vi "Actor Core.vi"(8 "error in":errorcluster, 11 "Nested in":refnum<class "MicroscopeController.lvclass">) -> (0 "error out":errorcluster, 3 "Actor out":refnum<class "Actor.lvclass">)   [LabVIEW 2020, in "MicroscopeController.lvlib" / "MicroscopeController.lvclass"]
doc: "(<B>Filename</B>: Actor Framework.lvlib:Actor.lvclass:Actor Core.vi)\n\nReceives messages to the actor, reacts to them, and initiates any error handling that may shut the actor down.\n\nDescendant classes may override this VI to append parallel tasks for the actor to complete while it handles messages. Overrides use the Call Parent Method node."
uses:
  MicroscopeController.lvclass
  C:/Program Files/National Instruments/LabVIEW 2020/vi.lib/ActorFramework/Actor/Actor.lvclass
  <vilib>/ActorFramework/Actor/Actor.lvclass
  MicroscopeController.lvclass/MicroscopeController.ctl
  <vilib>/ActorFramework/Actor/Actor.lvclass/Actor.ctl
  <vilib>/ActorFramework/Message Enqueuer/Message Enqueuer.lvclass/Message Enqueuer.ctl
  <vilib>/ActorFramework/Message Enqueuer/Init from Existing Queue.vi
  <vilib>/ActorFramework/Message Enqueuer/Enqueue.vi
  <vilib>/ActorFramework/Stop Msg/Stop Msg.lvclass
  C:/Program Files/National Instruments/LabVIEW 2020/vi.lib/ActorFramework/Message/Message.lvclass
  <vilib>/ActorFramework/Message Priority Queue/Priority Enqueue.vi
  <vilib>/ActorFramework/Message Enqueuer/Message Enqueuer.lvclass
  E:/Development/DevHardSoftware/MicroscopyFramework/ViewController/Microscope Controller/MicroscopeController.lvclass
  E:/Development/DevHardSoftware/MicroscopyFramework/Interface/DataListener/DataListener.lvclass
  E:/Development/DevHardSoftware/MicroscopyFramework/Interface/ErrorHandler/ErrorHandler.lvclass
panel:
  in  "Tab Control":T1(tab)
  out "SystemStatus":string
  # "https://sites.psu.edu/hancocklab/"
  # "Hancock Lab, The Pennsylvania State University.  email: woh1@psu.edu"
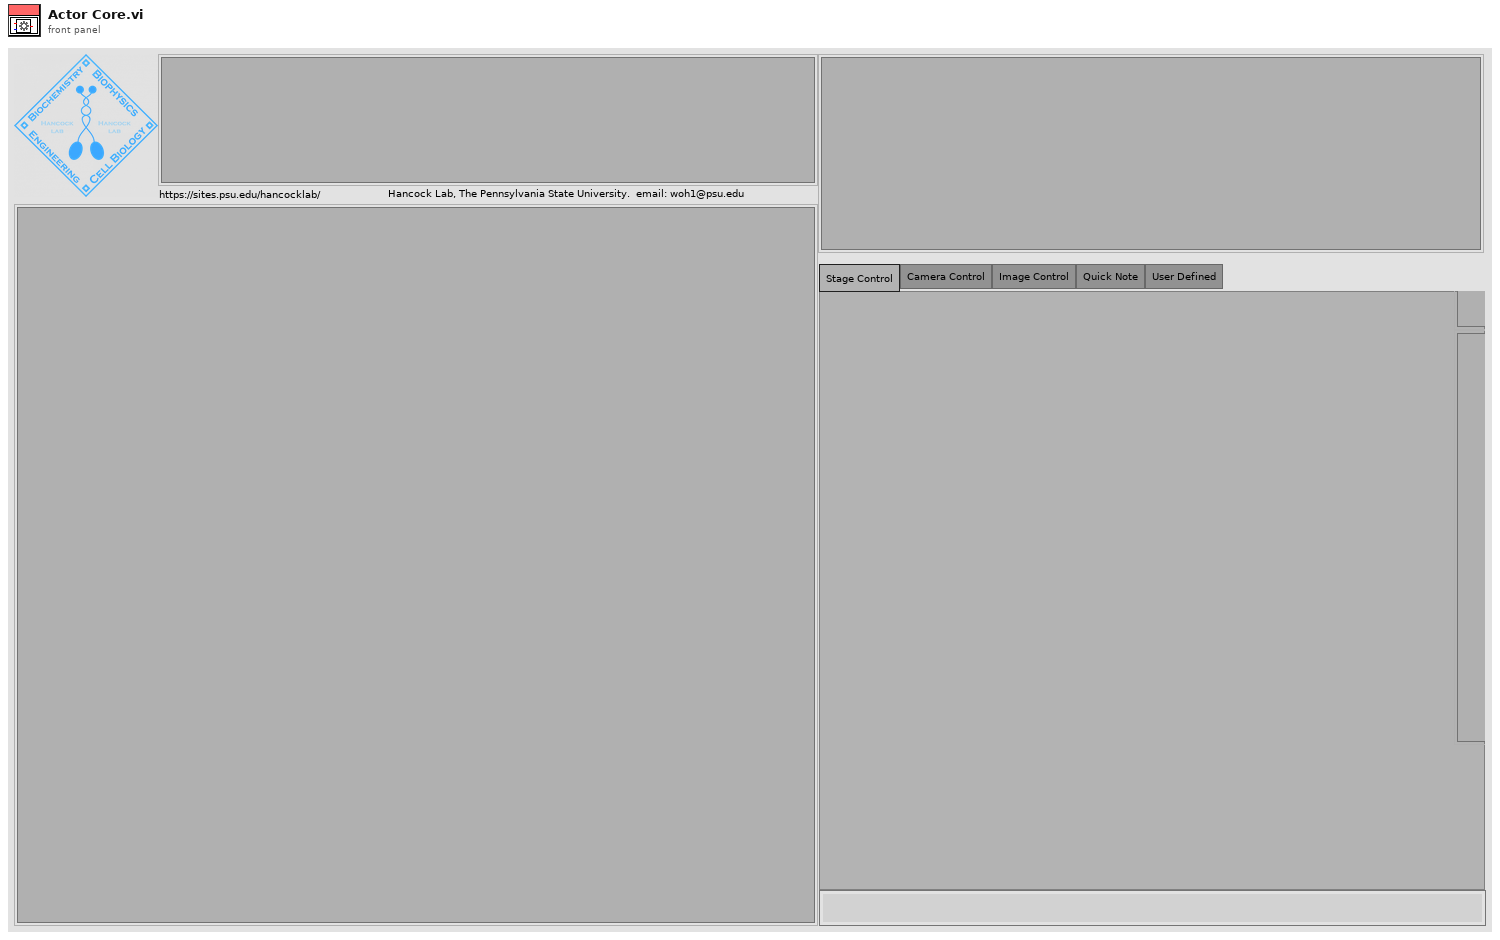
[diagram p1: front panel]
types:
  T1 = enum32{"Stage Control", "Camera Control", "Image Control", "Quick Note", "User Defined"}
  T2 = cluster{"Stop":refnum<user-event>, "SystemStatus":refnum<user-event>}
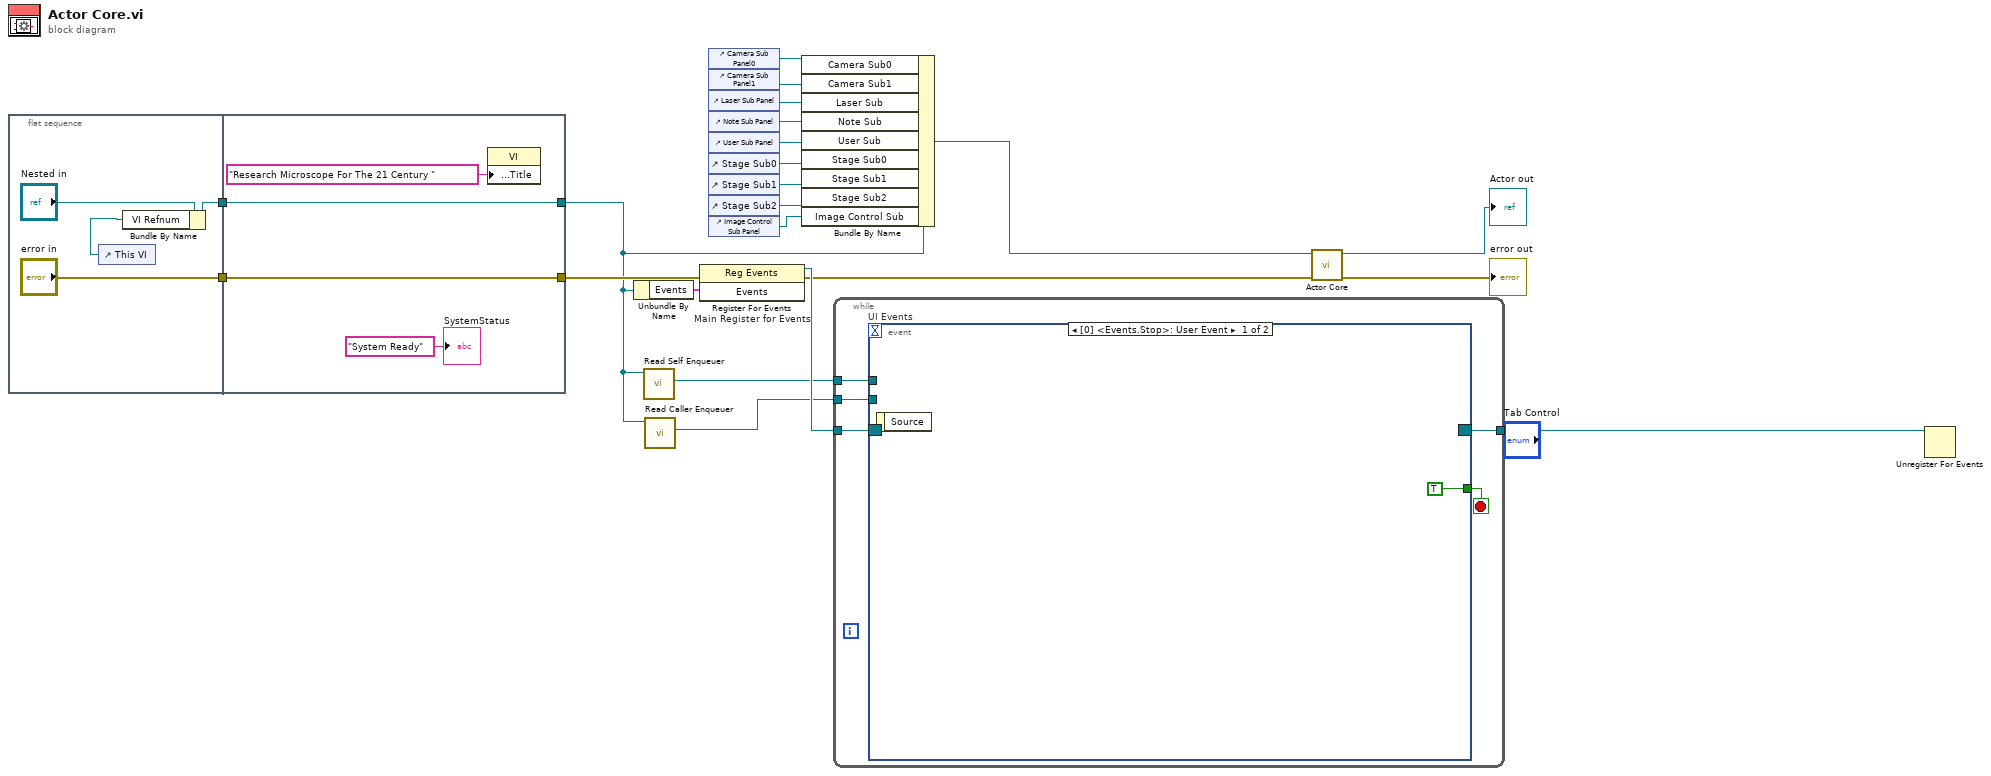
[diagram p0: block diagram]
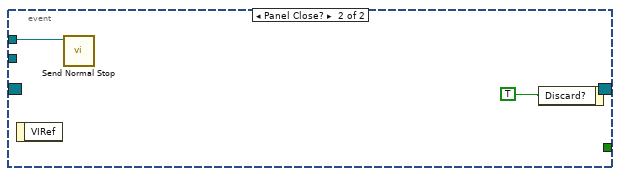
[diagram p2: hidden frame]
diagram:
  n1 = flat-sequence {
    tunnel: ["error in"] -> w2
    tunnel: [w24] -> w1
    tunnel: [w29] -> w4
    tunnel: [w30] -> w16
    tunnel: w2 -> [w30]
    tunnel: w1 -> [w29]
    frame #0 {
      n2 = control-ref of="This VI"() -> (w23:refnum<vi>)
      n3 = Bundle By Name(cluster="Nested in", "VI Refnum"=w23) -> (w24:refnum<class "MicroscopeController.lvclass">)
    }
    frame #1 {
      n4 = property class="VI"("Front Panel.Title"="Research Microscope For The 21 Century " ("Front Panel Window:Title")) -> ()  [unwired: 2 in, 2 out]
      "SystemStatus" <- "System Ready" ("SystemStatus")
    }
  }
  n5 = Unbundle By Name(w4) -> ("Events"=w19:T2)
  n6 = call <vilib>:"Read Self Enqueuer.vi"("Actor"=w4) -> ("Self Enqueuer"=w17:refnum<class "Message Enqueuer.lvclass">)  [unwired: 10 in]
  n7 = call <vilib>:"Read Caller Enqueuer.vi"("Actor"=w4) -> ("Caller Enqueuer"=w14:refnum<class "Message Enqueuer.lvclass">)  [unwired: 10 in]
  n8 = register-events "Main Register for Events"(error in=w16, w19) -> (reference out=w20:refnum<event-registration>, error out=w15:errorcluster)  [unwired: 1 in]
  n9 = control-ref of="Camera Sub Panel0"() -> (w6:refnum<vi>)
  n10 = control-ref of="Camera Sub Panel1"() -> (w12:refnum<vi>)
  n11 = control-ref of="Laser Sub Panel"() -> (w11:refnum<vi>)
  n12 = control-ref of="Note Sub Panel"() -> (w3:refnum<vi>)
  n13 = control-ref of="User Sub Panel"() -> (w10:refnum<vi>)
  n14 = control-ref of="Stage Sub0"() -> (w7:refnum<vi>)
  n15 = control-ref of="Stage Sub1"() -> (w9:refnum<vi>)
  n16 = control-ref of="Stage Sub2"() -> (w8:refnum<vi>)
  n17 = control-ref of="Image Control Sub Panel"() -> (w5:refnum<vi>)
  n18 = Bundle By Name(cluster=w4, "Camera Sub0"=w6, "Camera Sub1"=w12, "Laser Sub"=w11, "Note Sub"=w3, "User Sub"=w10, "Stage Sub0"=w7, "Stage Sub1"=w9, "Stage Sub2"=w8, "Image Control Sub"=w5) -> (w13:refnum<class "MicroscopeController.lvclass">)
  n19 = while {
    tunnel: w20 -> [w35]
    tunnel: [w33] -> w18
    tunnel: w17 -> [w32]
    tunnel: w14 -> [w31]
    stop <- w34 stop-if-true
    n20 = event "UI Events" shown="[0] <Events.Stop>: User Event" {
      selector: w35 -> [_ _]
      dyn-events: [_ _] -> w33
      timeout: _ -> [_ _]
      tunnel: [TRUE _] -> w34
      tunnel: w32 -> [_ w37]
      tunnel: w31 -> [_ _]
      event User Event {
        n21 = event-data() -> ()  [unwired: 1 in, 1 out]
      }
      event Panel Close? {
        n22 = event-data() -> ()  [unwired: 1 in, 1 out]
        n23 = call <vilib>:"Send Normal Stop.vi"("Message Enqueuer"=w37) -> ()  [unwired: 10 in, 1 out]
        n24 = event-data("Discard?"=TRUE) -> ()  [unwired: 1 in, 1 out]
      }
    }
  }
  n25 = call-parent "Actor Core.vi"("error in"=w15, "Actor in"=w13) -> ("error out"=→"error out":errorcluster, "Actor out"=→"Actor out":refnum<class "Actor.lvclass">)  [unwired: 8 in]
  n26 = Unregister For Events(event registration refnum=w18) -> ()  [unwired: 1 in, 1 out]
